vi "OAT Waterfall Plot.vi"(0 "spectral map":dbl[][](array[numeric]) format="%.2f", 1 "waterfall plot ref":refnum<vi>, 2 "reset? (F)":bool, 5 "spectral map info":T1={"scales"={"x scale"={"offset"=0.0, "multiplier"=0.0}, "y scale"={"offset"=0.0, "multiplier"=0.0}}, "unit labels"={"x-axis unit label"="", "y-axis unit label"="", "z-axis unit label"=""}, "plot type"=enum."Frequency-Time", "dB on"=TRUE} {"scales"."y scale"."multiplier" format="%.2f"; "scales"."y scale"."offset" format="%.2f"; "scales"."x scale"."multiplier" format="%.2f"; "scales"."x scale"."offset" format="%.2f"}, 9 "grids to display [Hz/Order]":dbl[](array[numeric]), 11 "error in (no error)":errorcluster, 12 "plot settings":T2={"plot color"=16860, "grid color"=11776947, "max Z range"=11, "number of spectra"=40} {"max Z range" items=["10^-7", "10^-6", "10^-5", "0.0001", "0.001", "0.01", "0.1", "1", "10", "100", "1000", "auto z range"]}) -> (4 "waterfall plot":T3, 15 "error out":errorcluster)   [LabVIEW 2017]
doc: "LabVIEW no longer supports this VI. Use the OAT Spectral Map VI instead. Receives the <B>spectral map</B> input from the OAT Spectral Map VI and continuously displays the spectral lines as a function of time in a waterfall plot."
uses:
  <vilib>/addons/Sound and Vibration/Order Analysis/Backward Compatibility/SubVIs/OAT Waterfall Plot.ctl
  <vilib>/addons/Sound and Vibration/Order Analysis/Resample Order Tracking/SubVIs/Spectral Map Info.ctl
  <vilib>/addons/Sound and Vibration/Order Analysis/Resample Order Tracking/SoundVib_Resampling.lvlib
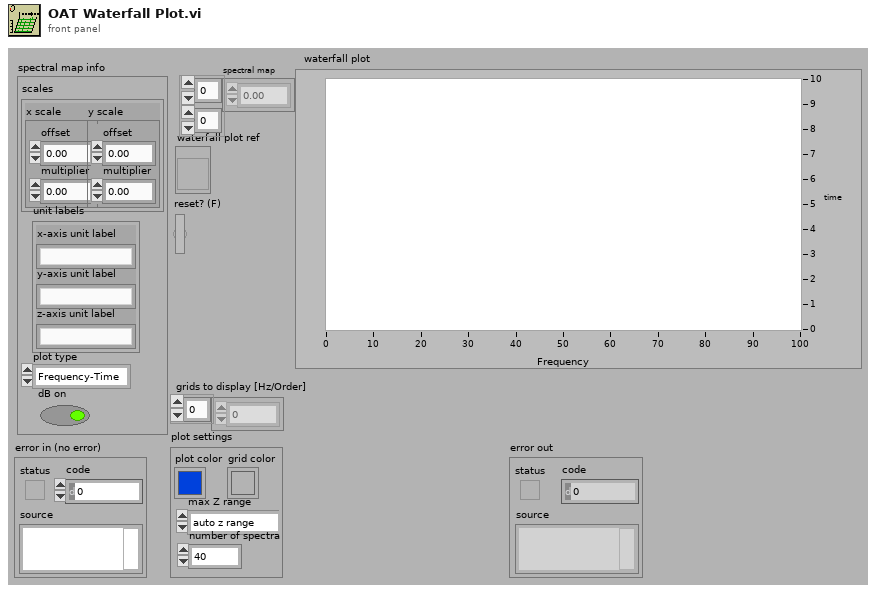
[diagram p1: front panel]
types:
  T1 = typedef "SoundVib_Resampling.lvlib/Spectral Map Info.ctl" = cluster{"scales":cluster{"x scale":cluster{"offset":dbl, "multiplier":dbl}, "y scale":cluster{"offset":dbl, "multiplier":dbl}}, "unit labels":cluster{"x-axis unit label":string, "y-axis unit label":string, "z-axis unit label":string}, "plot type":enum16{"Frequency-Time", "Time-Frequency", "Order-Time", "Time-Order", "Frequency-RPM", "RPM-Frequency", "Order-RPM", "RPM-Order"}, "dB on":bool}
  T2 = cluster{"plot color":u32, "grid color":u32, "max Z range":u16, "number of spectra":i32}
  T3 = typedef "OAT Waterfall Plot.ctl" = cluster{"X0":dbl, "dX":dbl, "Y":dbl[]}[]
  T4 = cluster{"x scale":cluster{"offset":dbl, "multiplier":dbl}, "y scale":cluster{"offset":dbl, "multiplier":dbl}}
  T5 = cluster{"x-axis unit label":string, "y-axis unit label":string, "z-axis unit label":string}
  T6 = enum16{"Frequency-Time", "Time-Frequency", "Order-Time", "Time-Order", "Frequency-RPM", "RPM-Frequency", "Order-RPM", "RPM-Order"}
  T7 = cluster{"plot color":u32, "grid color":u32, dbl, "max Z range":u16, "number of spectra":i32}
  T8 = cluster{"num of displayed spectra":i32, "num of new spectra":i32}
  T9 = cluster{"plot color":u32, "grid color":u32, "X shift (rel to total X)":dbl, "max Z range":u16, "number of spectra":i32}
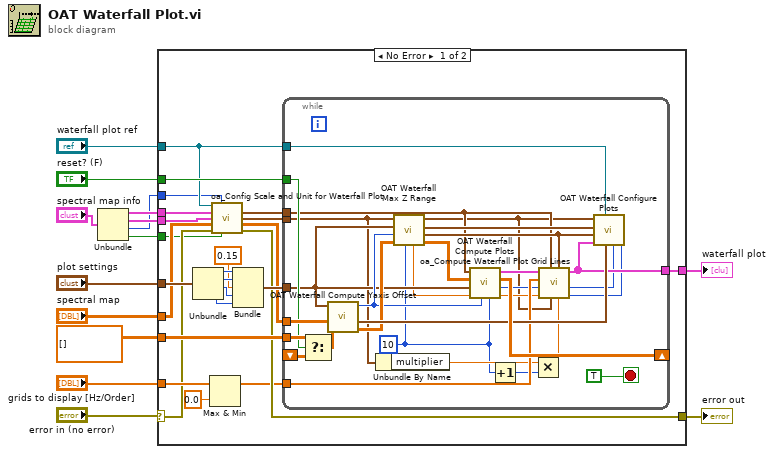
[diagram p0: block diagram]
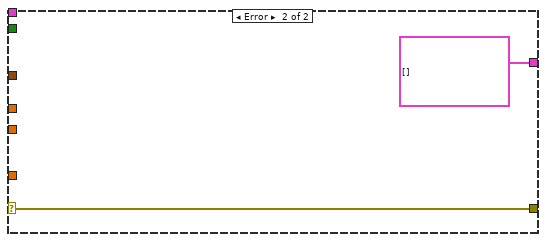
[diagram p2: hidden frame]
diagram:
  n1 = Unbundle("spectral map info") -> ("scales"=w4:T4, "unit labels"=w3:T5, "plot type"=w2:T6, "dB on"=w1:bool)
  n2 = case shown="No Error" "error in (no error)" {
    selector: "error in (no error)" -> [w19 w70]
    tunnel: w4 -> [w35 _]
    tunnel: "spectral map" -> [w23 _]
    tunnel: "reset? (F)" -> [w38 _]
    tunnel: dbl[][] [] -> [w37 _]
    tunnel: "plot settings" -> [w28 _]
    tunnel: "waterfall plot ref" -> [w34 _]
    tunnel: w3 -> [w32 _]
    tunnel: [w18 w70] -> w8
    tunnel: [w36 cluster{"X0":dbl, "dX":dbl, "Y":dbl[]}[] [] ("waterfall plot")] -> w7
    tunnel: w2 -> [w33 _]
    tunnel: "grids to display [Hz/Order]" -> [w29 _]
    tunnel: w1 -> [w17 _]
    frame No Error {
      n3 = Unbundle(w28) -> ("plot color"=w27:u32, "grid color"=w26:u32, "max Z range"=w21:u16, "number of spectra"=w20:i32)
      n4 = Max & Min(x=w29, y=0.0) -> (max(x,y)=w16:dbl[])  [unwired: 1 out]
      n5 = call <vilib>:"oa_Config Scale and Unit for Waterfall Plot.vi"("waterfall plot ref"=w34, "plot type"=w33, "scales"=w35, "unit labels"=w32, "spectral map"=w23, "error in (no error)"=w19, "dB on"=w17) -> ("X scale"=w30:cluster{"offset":dbl, "multiplier":dbl}, "Y scale"=w31:cluster{"offset":dbl, "multiplier":dbl}, "spectral map out"=w22:dbl[][], "error out"=w18:errorcluster)  [unwired: 5 in]
      n6 = Bundle("plot color"=w27, "grid color"=w26, 0.15, "max Z range"=w21, "number of spectra"=w20) -> (w25:T7)  [unwired: 1 in]
      n7 = while {
        shift-right: [w65] -> _
        shift-left: _ -> [w68]
        tunnel: w22 -> [w63]
        tunnel: w38 -> [w57]
        tunnel: w37 -> [w66]
        tunnel: w34 -> [w62]
        tunnel: [w55] -> w36
        tunnel: w31 -> [w46]
        tunnel: w30 -> [w47]
        tunnel: w16 -> [w52]
        tunnel: w25 -> [w48]
        stop <- TRUE stop-if-true
        w42 = 10 ("zoom factor")
        n8 = Select(t=w66, s=w57, f=w68) -> (s? t:f=w64:dbl[][])
        n9 = call <vilib>:"OAT Waterfall Compute Yaxis Offset.vi"("spectral map history"=w64, "spectral map new"=w63, "plot settings"=w48) -> ("spectral map for display"=w60:dbl[][], "spectra info"=w61:T8, "Y axis offset"=w54:i32)  [unwired: 6 in]
        n10 = Unbundle By Name(w46) -> ("multiplier"=w44:dbl)
        n11 = call <vilib>:"OAT Waterfall Max Z Range.vi"("zoom factor"=w42, "spectral map in"=w60, "Y axis offset"=w54, "plot settings"=w48, "scale in"=w46) -> ("spectral map out"=w59:dbl[][], "Y range"=w53:cluster{"min":dbl, "max":dbl}, "plot settings"=w58:T9, "scale out"=w41:cluster{"offset":dbl, "multiplier":dbl}, "max Z range"=w45:dbl)  [unwired: 2 in]
        n12 = call <vilib>:"OAT Waterfall Compute Plots.vi"("zoom factor"=w42, "Y axis offset"=w54, "max Z range"=w45, "plot settings"=w48, "spectral map in"=w59, "X scale"=w47) -> ("max x axis offset"=w51:dbl, "# of bins"=w50:i32, "spectral map out"=w65:dbl[][], "waterfall plot"=w56:cluster{"X0":dbl, "dX":dbl, "Y":dbl[]}[])  [unwired: 2 in]
        n13 = Increment(x=w42) -> (x+1=w40:i32)
        n14 = Multiply(x=w44, y=w40) -> (x*y=w43:dbl)
        n15 = call <vilib>:"oa_Compute Waterfall Plot Grid Lines.vi"("zoom factor"=w43, "Y range"=w53, "Y scale"=w41, "X scale"=w47, "max x axis offset"=w51, "# of bins"=w50, "grid lines to plot [Hz/Order]"=w52, "waterfall plot"=w56) -> ("# of axis lines"=w39:i32, "# of grid lines"=w49:i32, "waterfall plot out"=w55:cluster{"X0":dbl, "dX":dbl, "Y":dbl[]}[])  [unwired: 1 in]
        n16 = call <vilib>:"OAT Waterfall Configure Plots.vi"("# of axis lines"=w39, "# of grid lines"=w49, "spectra info"=w61, "reference"=w62, "waterfall plot"=w55, "Y range"=w53, "plot settings"=w58, "Y scale"=w41) -> ()  [unwired: 3 in, 1 out]
      }
    }
    frame Error {
    }
  }
  "error out" <- w8
  "waterfall plot" <- w7
